vi "TestExec.Config, Get Station SW Module Info.vi"(7 "Error if EXE does not exist":bool, 8 "Error if File Doesn't Exist":bool, 9 "Create File if Doesn't Exist":bool, 11 "Path":path=path "C:/MTE/Test Executive/Config") -> (0 "error out":errorcluster, 1 "Station IP Port":i32, 2 "Station Name":string, 3 "Sta Exe Path":path)   [LabVIEW 2018]
uses:
  <vilib>/Utility/config.llb/Read Key (String).vi
  <vilib>/Utility/config.llb/Read Key (I32).vi
  <vilib>/Utility/config.llb/Read Key (Path).vi
  <vilib>/KATE/Files/File Utils.lvlib
  <vilib>/Utility/config.llb/NI_LVConfig.lvlib
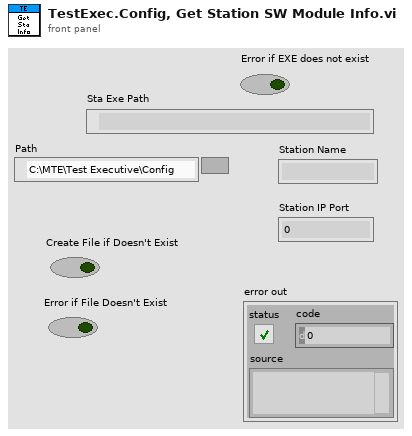
[diagram p1: front panel]
types:
  T1 = cluster{"Sta App":path, "Station Config":path, "ListenPort":u32, "Sta Name":string, "Station Folder":path}
  T2 = typedef "NI_LVConfig.lvlib/Config Data RefNum.ctl" = refnum<k1>
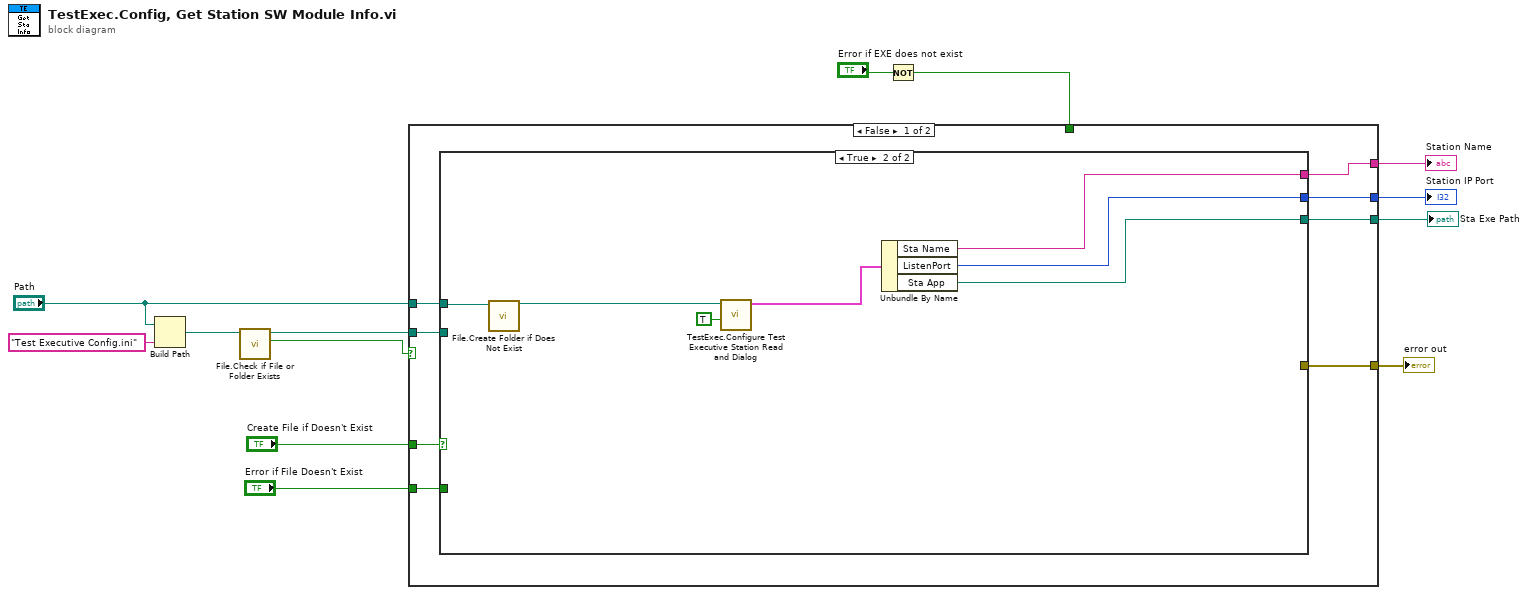
[diagram p0: block diagram]
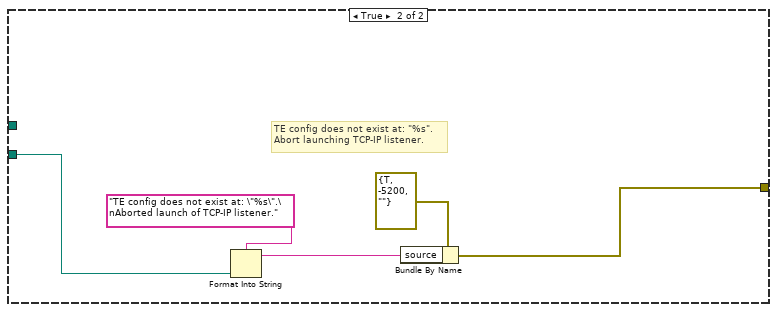
[diagram p3: hidden frame]
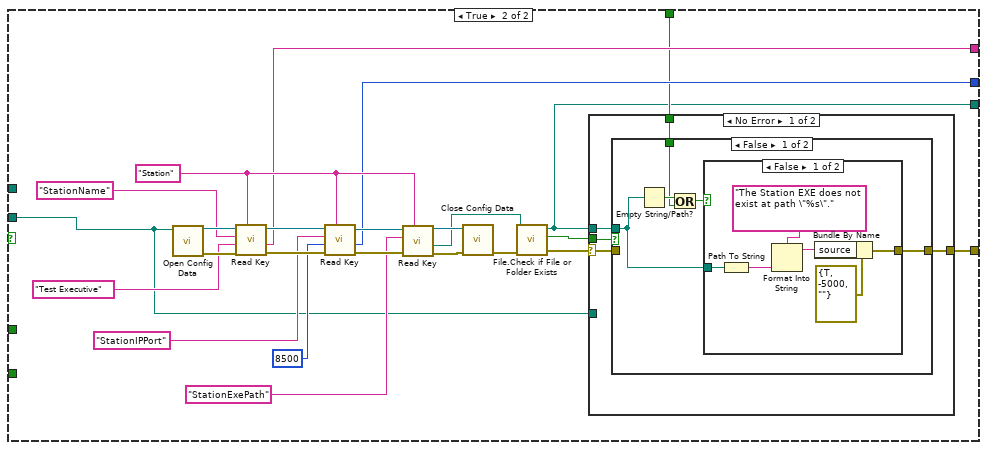
[diagram p4: hidden frame]
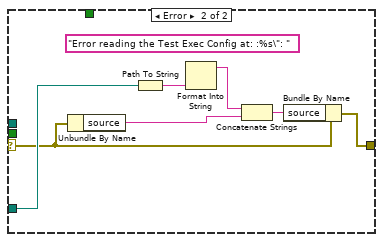
[diagram p7: hidden frame]
diagram:
  n1 = Build Path(base path="Path", name or relative path="Test Executive Config.ini") -> (appended path=w11:path)
  n2 = call <vilib>:"File.Check if File or Folder Exists.vi"("Path"=w11) -> ("Exists"=w9:bool, "Dup Path"=w10:path)  [unwired: 6 in, 3 out]
  n3 = Not(x="Error if EXE does not exist") -> (.not. x?=w2:bool)
  n4 = case shown="False" w9 {
    tunnel: [w21 w58] -> w13
    tunnel: w10 -> [w16 w42]
    tunnel: "Create File if Doesn't Exist" -> [w20 _]
    tunnel: [w18 w41] -> w7
    tunnel: [w19 w40] -> w6
    tunnel: "Error if File Doesn't Exist" -> [w17 _]
    tunnel: "Path" -> [w15 _]
    tunnel: w2 -> [_ w39]
    tunnel: [w14 w38] -> w1
    frame False {
      n5 = case shown="True" w20 {
        tunnel: [w23 _] -> w21
        tunnel: [_ w32] -> w19
        tunnel: [_ w33] -> w18
        tunnel: w17 -> [w25 _]
        tunnel: w16 -> [w24 _]
        tunnel: w15 -> [w22 w37]
        tunnel: [_ w31] -> w14
        frame False {
          n6 = case shown="False" w25 {
            tunnel: w24 -> [_ w29]
            tunnel: [_ w26] -> w23
            tunnel: w22 -> [_ _]
            frame False {
            }
            frame True {
              # "TE config does not exist at: \"%s\".\nAbort launching TCP-IP listener."
              n7 = Format Into String(format string="TE config does not exist at: \"%s\".\nAborted launch of TCP-IP listener." ("source"), w29) -> (resulting string=w27:string)  [unwired: 2 in, 1 out]
              n8 = Bundle By Name(cluster=errorcluster {"status"=TRUE, "code"=-5200, "source"=""} ("error constant"), "source"=w27) -> (w26:errorcluster)
            }
          }
        }
        frame True {
          n9 = call <vilib>:"File.Create Folder if Does Not Exist.vi"("Path"=w37) -> ("Dup Path"=w36:path)  [unwired: 8 in, 2 out]
          n10 = call "TestExec.Configure Test Executive Station Read and Dialog.vi"("Dialog"=TRUE, "TE Config Folder"=w36) -> ("Config Out"=w34:T1)  [unwired: 8 in, 1 out]
          n11 = Unbundle By Name(w34) -> ("Sta Name"=w33:string, "ListenPort"=w32:u32, "Sta App"=w31:path)
        }
      }
    }
    frame True {
      w48 = "Station" ("section")
      n12 = call <vilib>:"Open Config Data.vi"("configuration file path"=w42) -> ("error out"=w56:errorcluster, "refnum"=w57:T2)  [unwired: 8 in, 1 out]
      n13 = call-poly <vilib>:"Read Key.vi"("section"=w48, "error in (no error)"=w56, "default value"="Test Executive" ("section"), "key"="StationName" ("section"), "refnum"=w57) -> ("error out"=w55:errorcluster, "value"=w41:string, "refnum out"=w54:T2)  [unwired: 3 in, 1 out]
      n14 = call-poly <vilib>:"Read Key.vi"("section"=w48, "error in (no error)"=w55, "default value"=8500, "key"="StationIPPort", "refnum"=w54) -> ("error out"=w51:errorcluster, "value"=w40:i32, "refnum out"=w52:T2)  [unwired: 3 in, 1 out]
      n15 = call-poly <vilib>:"Read Key.vi"("section"=w48, "error in (no error)"=w51, "key"="StationExePath", "refnum"=w52) -> ("error out"=w50:errorcluster, "value"=w44:path, "refnum out"=w49:T2)  [unwired: 4 in, 1 out]
      n16 = call <vilib>:"Close Config Data.vi"("error in (no error)"=w50, "refnum"=w49) -> ("error out"=w61:errorcluster)  [unwired: 8 in, 1 out]
      n17 = call <vilib>:"File.Check if File or Folder Exists.vi"("error in"=w61, "Path"=w44) -> ("error out"=w60:errorcluster, "Exists"=w59:bool, "Dup Path"=w38:path)  [unwired: 5 in, 2 out]
      n18 = case shown="No Error" w60 {
        selector: w60 -> [w64 w80]
        tunnel: w59 -> [w66 _]
        tunnel: w38 -> [w65 _]
        tunnel: [w63 w79] -> w58
        tunnel: w42 -> [_ w84]
        tunnel: w39 -> [w62 _]
        frame No Error {
          n19 = case shown="False" w66 {
            tunnel: w65 -> [w70 _]
            tunnel: w64 -> [_ w78]
            tunnel: [w71 w78] -> w63
            tunnel: w62 -> [w67 _]
            frame False {
              n20 = Empty String/Path?(string/path=w70) -> (empty?=w69:bool)
              n21 = Or(x=w69, y=w67) -> (x .or. y?=w68:bool)
              n22 = case shown="False" w68 {
                tunnel: [w73 _] -> w71
                tunnel: w70 -> [w72 _]
                frame False {
                  n23 = Path To String(path=w72) -> (string=w77:string)
                  n24 = Format Into String(format string="The Station EXE does not exist at path \"%s\".", w77) -> (resulting string=w75:string)  [unwired: 2 in, 1 out]
                  n25 = Bundle By Name(cluster=errorcluster {"status"=TRUE, "code"=-5000, "source"=""} ("error constant"), "source"=w75) -> (w73:errorcluster)
                }
                frame True {
                }
              }
            }
            frame True {
            }
          }
        }
        frame Error {
          (unwired) "Error reading the Test Exec Config at: :%s\": "
          n26 = Unbundle By Name(w80) -> ("source"=w82:string)
          n27 = Path To String(path=w84) -> (string=w85:string)
          n28 = Format Into String(w85) -> (resulting string=w83:string)  [unwired: 3 in, 1 out]
          n29 = Concatenate Strings(w83, w82) -> (w81:string)
          n30 = Bundle By Name(cluster=w80, "source"=w81) -> (w79:errorcluster)
        }
      }
    }
  }
  "error out" <- w13
  "Station Name" <- w7
  "Station IP Port" <- w6
  "Sta Exe Path" <- w1
